vi "Auton scroll.vi"(1 "Down 1":bool, 2 "Up 1":bool) -> (0 "Numeric":i32)   [LabVIEW 2013]
uses:
  <vilib>/Rock Robotics/WPI/DriverStation/DriverStationLCD/WPI_DriverStationLCDLCDLine.ctl
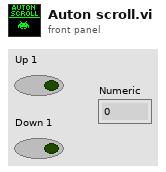
[diagram p1: front panel]
types:
  T1 = typedef "WPI_DriverStationLCDLCDLine.ctl" = enum16{"Main - Line 1", "User - Line 2", "User - Line 3", "User - Line 4", "User - Line 5", "User - Line 6"}
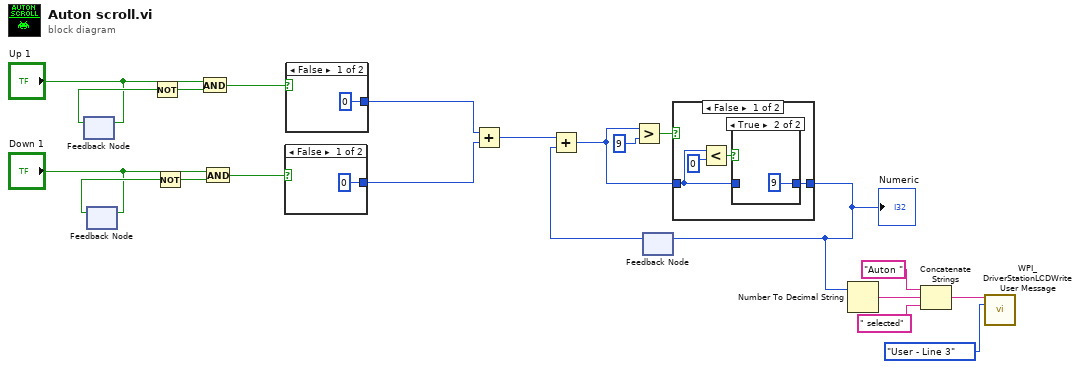
[diagram p0: block diagram]
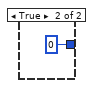
[diagram p3: hidden frame]
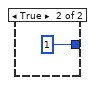
[diagram p4: hidden frame]
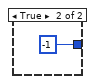
[diagram p5: hidden frame]
diagram:
  n1 = feedback #1() -> (w20:bool)  [unwired: 1 in]
  n2 = feedback-in #1("Up 1") -> ()
  n3 = feedback #2() -> (w19:bool)  [unwired: 1 in]
  n4 = feedback-in #2("Down 1") -> ()
  n5 = Not(x=w20) -> (.not. x?=w21:bool)
  n6 = Not(x=w19) -> (.not. x?=w18:bool)
  n7 = And(x="Up 1", y=w21) -> (x .and. y?=w17:bool)
  n8 = And(x="Down 1", y=w18) -> (x .and. y?=w16:bool)
  n9 = case shown="False" w16 {
    tunnel: [0 1] -> w6
    frame False {
    }
    frame True {
    }
  }
  n10 = case shown="False" w17 {
    tunnel: [0 -1] -> w5
    frame False {
    }
    frame True {
    }
  }
  n11 = Add(x=w5, y=w6) -> (x+y=w15:i32)
  n12 = feedback #3() -> (w14:i32)  [unwired: 1 in]
  n13 = Add(x=w15, y=w14) -> (x+y=w12:i32)
  n14 = Greater?(x=w12, y=9) -> (0:w13:bool)
  n15 = case shown="False" w13 {
    tunnel: w12 -> [w28 _]
    tunnel: [w26 0] -> w4
    frame False {
      n16 = Less?(x=w28, y=0) -> (x < y?=w29:bool)
      n17 = case shown="True" w29 {
        tunnel: w28 -> [w30 _]
        tunnel: [w30 9] -> w26
        frame False {
        }
        frame True {
        }
      }
    }
    frame True {
    }
  }
  "Numeric" <- w4
  n18 = feedback-in #3(w4) -> ()
  n19 = Number To Decimal String(number=w4) -> (decimal integer string=w11:string)  [unwired: 1 in]
  n20 = Concatenate Strings("Auton " ("string"), w11, " selected" ("string")) -> (w8:string)
  n21 = call <vilib>:"WPI_DriverStationLCDWrite User Message.vi"("line text"=w8, "line"=WPI_DriverStationLCDLCDLine."User - Line 3") -> ()  [unwired: 13 in, 1 out]
